vi "CorrectDistance.vi"(0 "JoyStick 1":dbl format="%#_13g", 1 "JoyStick 2":dbl format="%#_13g", 3 "CenterPoint":dbl format="%#_13g", 4 "Range":dbl format="%#_13g", 5 "Distance":dbl format="%#_13g", 7 "Button":bool=TRUE) -> (21 "Right Motor":dbl format="%#_13g", 22 "Left Motor":dbl format="%#_13g", 23 "Less than":bool, 24 "Greater":bool, 25 "In Range?":bool, 26 "number":u32)   [LabVIEW 2016]
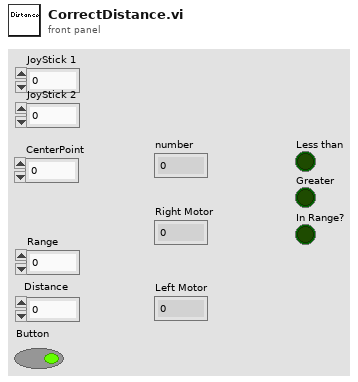
[diagram p1: front panel]
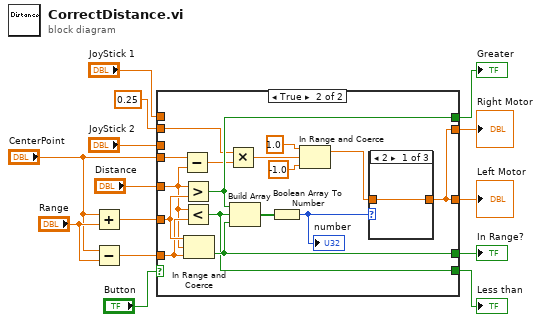
[diagram p0: block diagram]
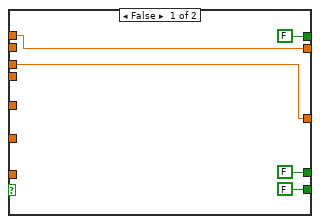
[diagram p2: hidden frame]
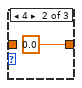
[diagram p3: hidden frame]
diagram:
  n1 = Add(x="CenterPoint", y="Range") -> (x+y=w13:dbl)
  n2 = Subtract(x="CenterPoint", y="Range") -> (x-y=w12:dbl)
  n3 = case shown="True" "Button" {
    tunnel: "JoyStick 1" -> [w19 _]
    tunnel: "JoyStick 2" -> [w18 _]
    tunnel: "Distance" -> [_ w20]
    tunnel: w13 -> [_ w34]
    tunnel: w12 -> [_ w27]
    tunnel: [w18 w29] -> w7
    tunnel: [w19 w29] -> w8
    tunnel: [FALSE w32] -> w6
    tunnel: [FALSE w31] -> w5
    tunnel: [FALSE w30] -> w4
    tunnel: "CenterPoint" -> [_ w28]
    tunnel: 0.25 -> [_ w25]
    frame False {
    }
    frame True {
      n4 = Subtract(x=w28, y=w20) -> (x-y=w26:dbl)
      n5 = Greater?(x=w20, y=w34) -> (0:w32:bool)
      n6 = Less?(x=w20, y=w27) -> (x < y?=w30:bool)
      n7 = In Range and Coerce(upper limit=w34, x=w20, lower limit=w27) -> (In Range?=w31:bool)  [unwired: 1 out]
      n8 = Multiply(x=w25, y=w26) -> (x*y=w24:dbl)
      n9 = Build Array(w32, w30, w31) -> (w33:bool[])
      n10 = Boolean Array To Number(Boolean array=w33) -> (number=w35:u32)
      "number" <- w35
      n11 = In Range and Coerce(upper limit=1.0, x=w24, lower limit=-1.0) -> (coerced(x)=w21:dbl)  [unwired: 1 out]
      n12 = case shown="2" w35 {
        tunnel: [w36 0.0 w38] -> w29
        tunnel: w21 -> [w36 _ w38]
        frame 2 {
        }
        frame 4 {
        }
        frame 1, Default {
        }
      }
    }
  }
  "Right Motor" <- w8
  "Left Motor" <- w7
  "Greater" <- w6
  "In Range?" <- w5
  "Less than" <- w4
